vi "Set PWM Frequency.vi"(8 "error in (no error)":errorcluster, 9 "frequency":u16, 11 "Grove I2C L298P Motor Drive in":refnum<class "Grove I2C L298P Motor Drive.lvclass">) -> (0 "error out":errorcluster, 3 "Grove I2C L298P Motor Drive out":refnum<class "Grove I2C L298P Motor Drive.lvclass">)   [LabVIEW 2020, in "CTI-Peripheral.lvlib" / "Grove I2C L298P Motor Drive.lvclass"]
uses:
  Grove I2C L298P Motor Drive.lvclass
  Grove I2C L298P Motor Drive.lvclass/Grove I2C L298P Motor Drive.ctl
  CTI/I2C Connection/I2C Connection.lvclass/I2C Connection.ctl
  CTI/Session/I2C Write Data.vi
  CTI/I2C Connection/I2C Connection.lvclass
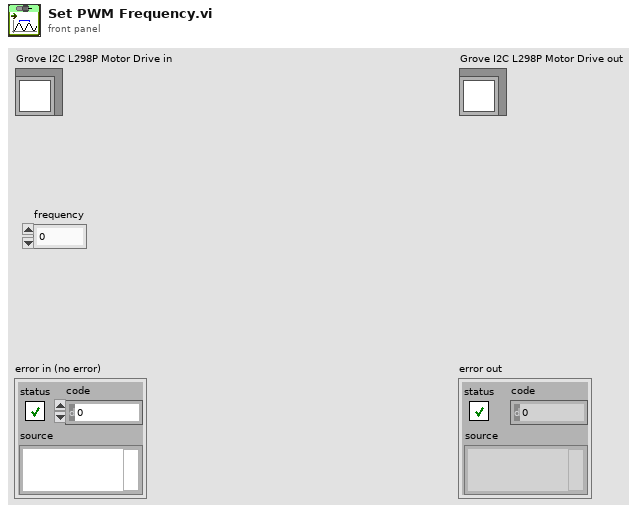
[diagram p1: front panel]
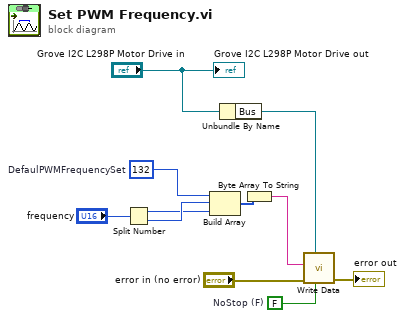
[diagram p0: block diagram]
diagram:
  w1 = u8 132  # DefaulPWMFrequencySet
  w8 = FALSE  # NoStop (F)
  n1 = Split Number(x="frequency") -> (hi(x)=w6:u8, lo(x)=w7:u8)
  n2 = Build Array(w1, w7, w6) -> (w5:u8[])
  n3 = Unbundle By Name("Grove I2C L298P Motor Drive in") -> ("Bus"=w9:refnum<class "I2C Connection.lvclass">)
  n4 = Byte Array To String(unsigned byte array=w5) -> (string=w3:string)
  n5 = call "Write Data.vi"("NoStop (F)"=w8, "I2C Connection"=w9, "error in (no error)"="error in (no error)", "Data"=w3) -> ("error out"=→"error out":errorcluster)  [unwired: 7 in]
  "Grove I2C L298P Motor Drive out" <- "Grove I2C L298P Motor Drive in"
